vi "example_02_xy_graph_scrollbar.vi"() -> ()   [LabVIEW 2015, in "lv-graph.lvlib"]
doc: "This example will generate a fixed number of points, and then allow navigation of the data using the hofizontal and vertical scrollbar. You can configure the data rate (how often data is generated) and the refresh rate (how often the graphs update). This is a working example of how to separate data generation from display."
uses:
  advanced/build_graph-single_axis.vi
  advanced/build_graph-vertical.vi
  lv-graph.lvlib
panel:
  in  "vertical_scrollbar":i32(c297)
  out "vertical_graph":T1(graph)
  in  "refresh":bool
  in  "Flipped?":bool
  in  "# of Points to Generate":i32=5000
  in  "Realtime?":bool
  out "all_points_generated":bool
  in  "horizontal_scrollbar":i32(c297)
  in  "data_rate_ms":u32=10
  in  "refresh_rate_ms":i32=250
  in  "stop":bool
  out "horizontal_graph":T2(graph)
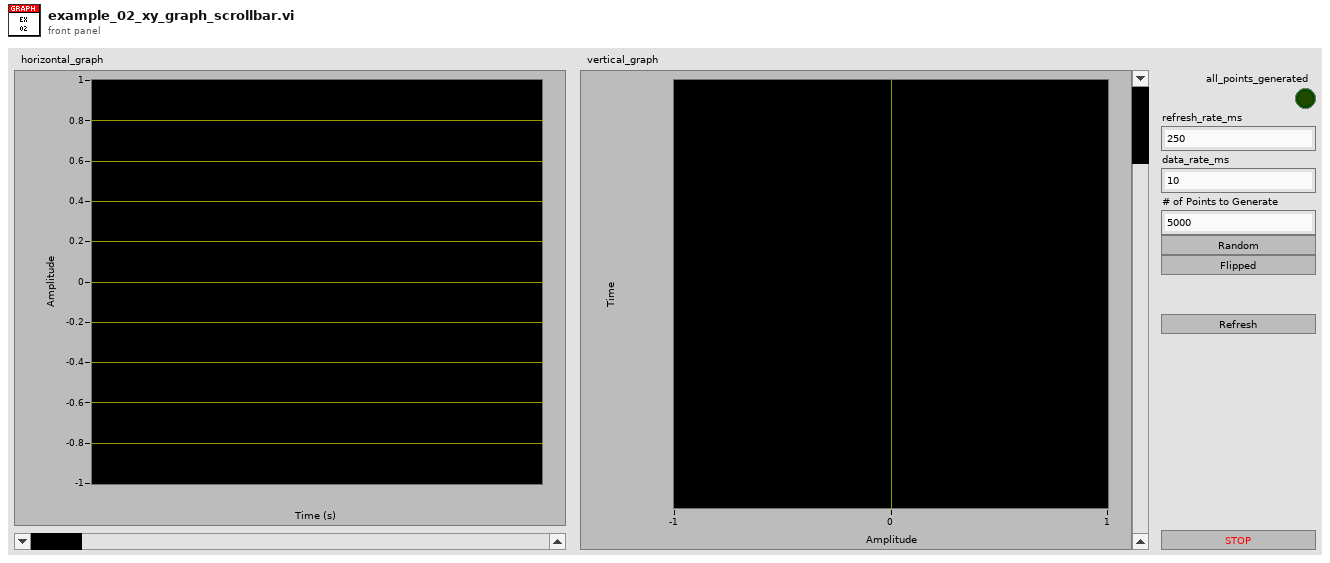
[diagram p1: front panel]
types:
  T1 = cluster{cluster{"Timestamp":dbl, "Timestamp":dbl}[]}[]
  T2 = cluster{"Time [] out":dbl[], "Data[][] out":dbl[]}[]
  T3 = cluster{"index":i32, "x_axis":dbl[], "y_axis":dbl[][]}
  T4 = cluster{"x_scale_maximum":dbl, "x_scale_minimum":dbl, "y_scale_maximum":dbl, "y_scale_minimum":dbl}
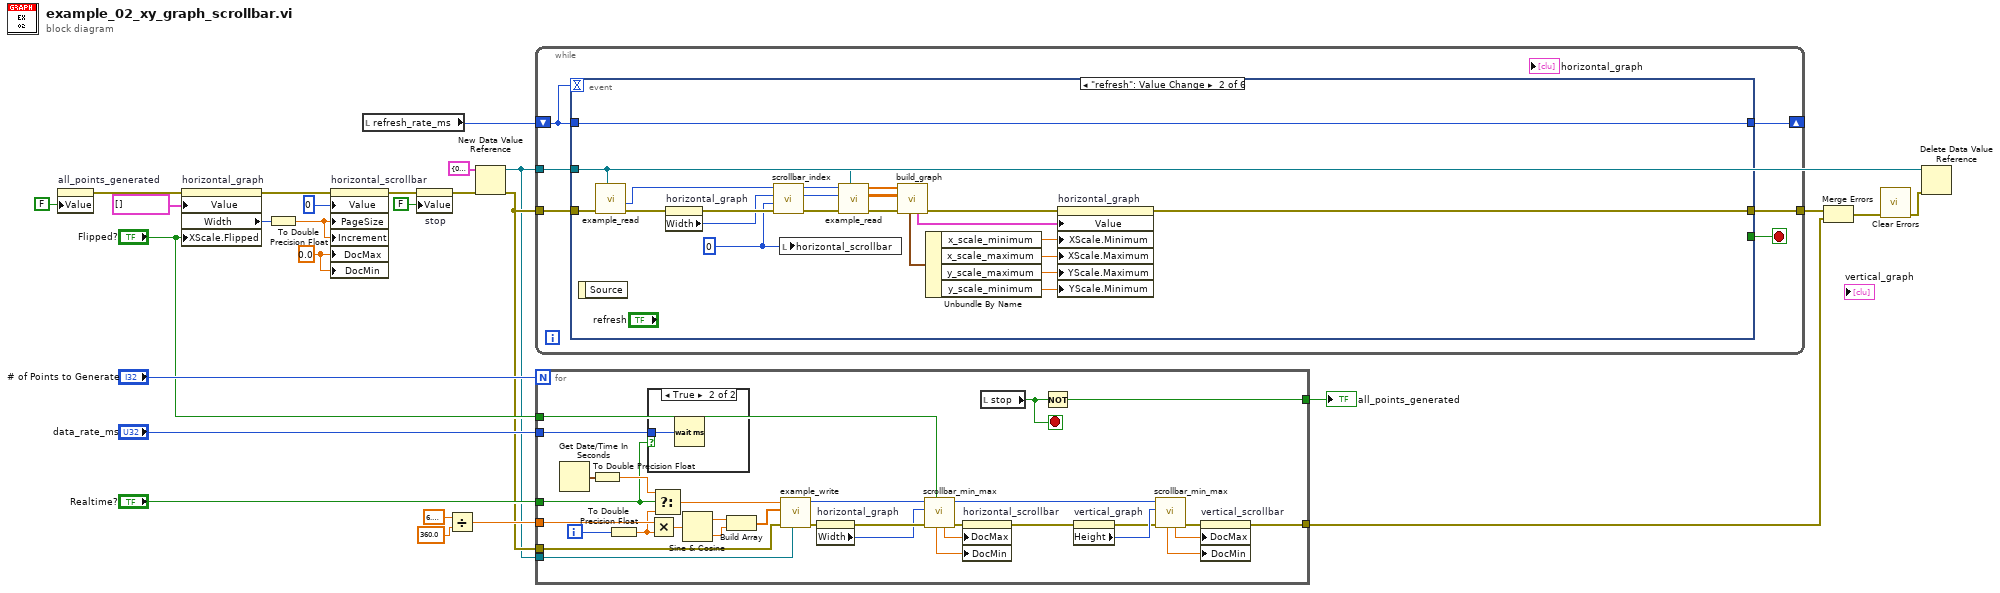
[diagram p0: block diagram]
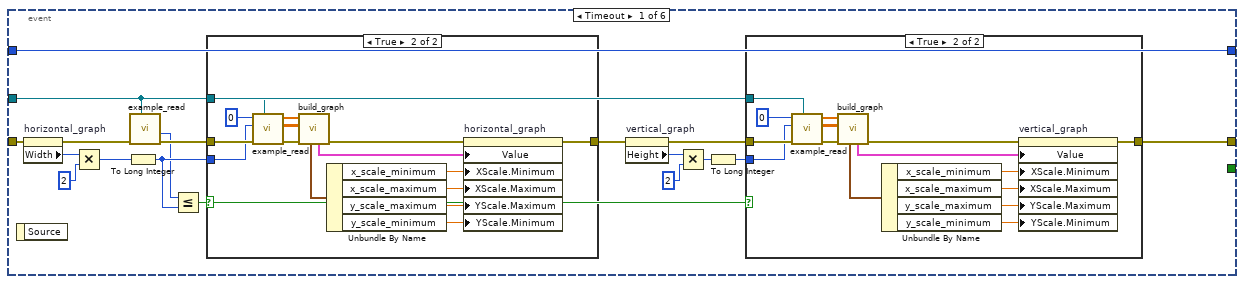
[diagram p2: hidden frame]
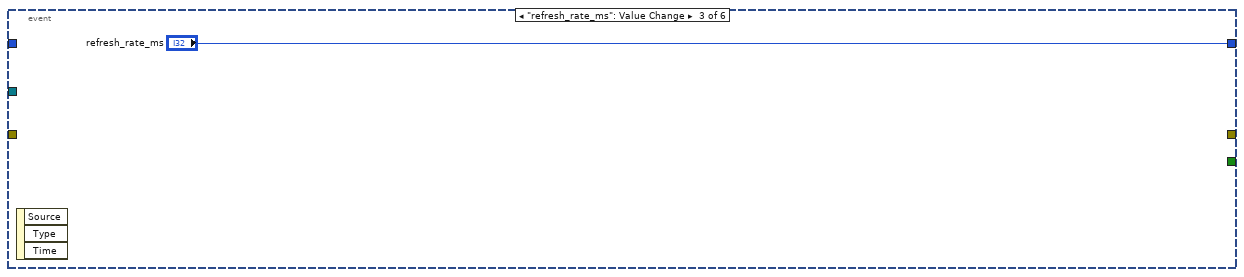
[diagram p5: hidden frame]
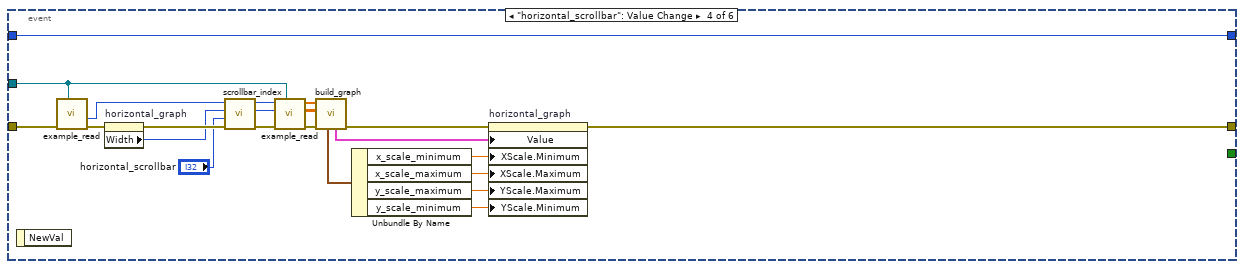
[diagram p6: hidden frame]
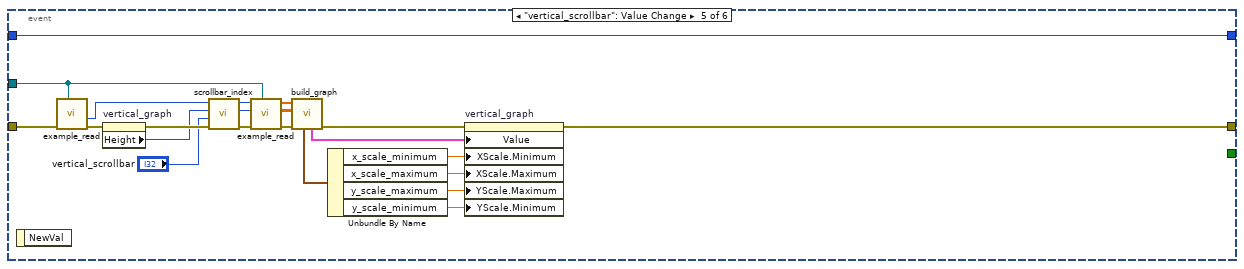
[diagram p7: hidden frame]
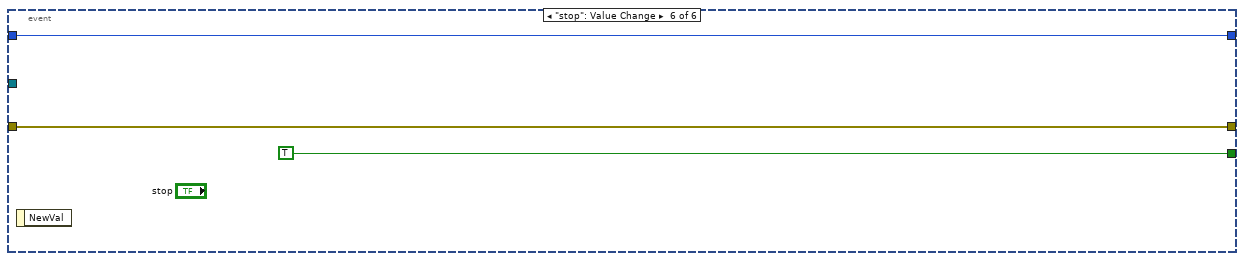
[diagram p8: hidden frame]
diagram:
  w18 = 0.0 ("Doc Max")
  n1 = property on="all_points_generated" class="Bool (strict)"("Value"=FALSE ("All Points Generated?")) -> (error out=w8:errorcluster)  [unwired: 2 in, 1 out]
  n2 = property on="horizontal_graph" class="XYGraph (strict)"(error in=w8, "Value"=T2 [] ("Graph"), "XScale.Flipped"="Flipped?") -> (error out=w19:errorcluster, "Width"=w17:u32)  [unwired: 1 in, 1 out]
  n3 = To Double Precision Float(number=w17) -> (double precision float=w6:dbl)
  n4 = property on="horizontal_scrollbar" class="Scroll (strict)"(error in=w19, "Value"=0 ("Scrollbar"), "PageSize"=w6, "Increment"=w6, "DocMax"=w18, "DocMin"=w18) -> (error out=w20:errorcluster)  [unwired: 1 in, 1 out]
  n5 = local read "refresh_rate_ms"() -> (w4:i32)
  n6 = property on="stop" class="Bool (strict)"(error in=w20, "Value"=FALSE ("Stop")) -> (error out=w26:errorcluster)  [unwired: 1 in, 1 out]
  n7 = Divide(x=6.283185307179586, y=360.0) -> (x/y=w12:dbl)
  n8 = New Data Value Reference(data value=T3 {"index"=0, "x_axis"=[], "y_axis"=[]} ("cluster"), error in=w26) -> (data value reference=w1:refnum<data-value>, error out=w3:errorcluster)
  n9 = while {
    tunnel: w3 -> [w33]
    tunnel: [w31] -> w25
    tunnel: w1 -> [w30]
    shift-right: [w28] -> _
    shift-left: w4 -> [w29]
    stop <- w32 stop-if-true
    n10 = event shown="[1] \"refresh\": Value Change" {
      selector: _ -> [_ _ _ _ _ _]
      dyn-events: _ -> [_ _ _ _ _ _]
      timeout: w29 -> [_ _ _ _ _ _]
      tunnel: w33 -> [w49 w101 _ w124 w146 w152]
      tunnel: [_ _ _ _ _ TRUE] -> w32
      tunnel: [w38 w105 _ w123 w145 w152] -> w31
      tunnel: w30 -> [w37 w94 _ w117 w140 _]
      tunnel: w29 -> [w44 w95 _ w119 w141 w151]
      tunnel: [w44 w95 "refresh_rate_ms" w119 w141 w151] -> w28
      event Timeout {
        n11 = event-data() -> ()  [unwired: 1 in, 1 out]
        n12 = property on="horizontal_graph" class="XYGraph (strict)"(error in=w49) -> (error out=w47:errorcluster, "Width"=w50:u32)  [unwired: 1 in, 1 out]
        n13 = Multiply(x=w50, y=u32 2 ("x")) -> (x*y=w48:u32)
        n14 = To Long Integer(number=w48) -> (32bit integer=w45:i32)
        n15 = call "example_read.vi"("dvr"=w37, "error in (no error)"=w47) -> ("error out"=w46:errorcluster, "index"=w35:i32)  [unwired: 6 in, 2 out]
        n16 = Less Or Equal?(x=w35, y=w45) -> (x <= y?=w34:bool)
        n17 = case shown="True" w34 {
          tunnel: w46 -> [w68 w78]
          tunnel: [w68 w75] -> w39
          tunnel: w45 -> [_ w73]
          tunnel: w37 -> [_ w76]
          frame False {
          }
          frame True {
            n18 = call "example_read.vi"("dvr"=w76, "error in (no error)"=w78, "length"=w73, "index in"=0 ("Index in")) -> ("error out"=w77:errorcluster, "y_axis"=w71:dbl[][], "x_axis"=w72:dbl[])  [unwired: 4 in, 1 out]
            n19 = call-poly "build_graph.vi"("error in (no error)"=w77, "y_axis"=w71, "x_axis"=w72) -> ("error out"=w83:errorcluster, "graph_data"=w69:cluster{dbl[], dbl[]}[], "scale_ranges"=w70:T4)  [unwired: 6 in]
            n20 = Unbundle By Name(w70) -> ("x_scale_minimum"=w81:dbl, "x_scale_maximum"=w82:dbl, "y_scale_maximum"=w80:dbl, "y_scale_minimum"=w79:dbl)
            n21 = property on="horizontal_graph" class="XYGraph (strict)"(error in=w83, "Value"=w69, "XScale.Minimum"=w81, "XScale.Maximum"=w82, "YScale.Maximum"=w80, "YScale.Minimum"=w79) -> (error out=w75:errorcluster)  [unwired: 1 in, 1 out]
          }
        }
        n22 = property on="vertical_graph" class="XYGraph (strict)"(error in=w39) -> (error out=w36:errorcluster, "Height"=w41:u32)  [unwired: 1 in, 1 out]
        n23 = Multiply(x=w41, y=u32 2 ("x")) -> (x*y=w42:u32)
        n24 = To Long Integer(number=w42) -> (32bit integer=w43:i32)
        n25 = case shown="True" w34 {
          tunnel: w36 -> [w52 w66]
          tunnel: [w52 w63] -> w38
          tunnel: w43 -> [_ w61]
          tunnel: w37 -> [_ w60]
          frame False {
          }
          frame True {
            n26 = call "example_read.vi"("dvr"=w60, "error in (no error)"=w66, "length"=w61, "index in"=0 ("Index in")) -> ("error out"=w65:errorcluster, "y_axis"=w64:dbl[][], "x_axis"=w59:dbl[])  [unwired: 4 in, 1 out]
            n27 = call-poly "build_graph.vi"("error in (no error)"=w65, "y_axis"=w64, "x_axis"=w59) -> ("error out"=w67:errorcluster, "graph_data"=w57:T1, "scale_ranges"=w58:T4)  [unwired: 6 in]
            n28 = Unbundle By Name(w58) -> ("x_scale_minimum"=w56:dbl, "x_scale_maximum"=w55:dbl, "y_scale_maximum"=w54:dbl, "y_scale_minimum"=w53:dbl)
            n29 = property on="vertical_graph" class="XYGraph (strict)"(error in=w67, "Value"=w57, "XScale.Minimum"=w56, "XScale.Maximum"=w55, "YScale.Maximum"=w54, "YScale.Minimum"=w53) -> (error out=w63:errorcluster)  [unwired: 1 in, 1 out]
          }
        }
      }
      event "refresh": Value Change {
        w100 = 0 ("Seek")
        n30 = event-data() -> ()  [unwired: 1 in, 1 out]
        n31 = call "example_read.vi"("dvr"=w94, "error in (no error)"=w101) -> ("error out"=w102:errorcluster, "index"=w88:i32)  [unwired: 6 in, 2 out]
        n32 = property on="horizontal_graph" class="XYGraph (strict)"(error in=w102) -> (error out=w104:errorcluster, "Width"=w103:u32)  [unwired: 1 in, 1 out]
        n33 = call "scrollbar_index.vi"("error in (no error)"=w104, "seek"=w100, "width_height"=w103, "data_available"=w88) -> ("error out"=w96:errorcluster, "length"=w89:i32, "index"=w90:i32)  [unwired: 5 in]
        n34 = local write "horizontal_scrollbar"(w100) -> ()
        n35 = call "example_read.vi"("dvr"=w94, "error in (no error)"=w96, "length"=w89, "index in"=w90) -> ("error out"=w97:errorcluster, "y_axis"=w98:dbl[][], "x_axis"=w91:dbl[])  [unwired: 4 in, 1 out]
        n36 = call-poly "build_graph.vi"("error in (no error)"=w97, "y_axis"=w98, "x_axis"=w91) -> ("error out"=w99:errorcluster, "graph_data"=w92:cluster{dbl[], dbl[]}[], "scale_ranges"=w93:T4)  [unwired: 6 in]
        n37 = Unbundle By Name(w93) -> ("x_scale_minimum"=w87:dbl, "x_scale_maximum"=w86:dbl, "y_scale_maximum"=w85:dbl, "y_scale_minimum"=w84:dbl)
        n38 = property on="horizontal_graph" class="XYGraph (strict)"(error in=w99, "Value"=w92, "XScale.Minimum"=w87, "XScale.Maximum"=w86, "YScale.Maximum"=w85, "YScale.Minimum"=w84) -> (error out=w105:errorcluster)  [unwired: 1 in, 1 out]
      }
      event "refresh_rate_ms": Value Change {
        n39 = event-data() -> ()  [unwired: 1 in, 3 out]
      }
      event "horizontal_scrollbar": Value Change {
        n40 = event-data() -> ()  [unwired: 1 in, 1 out]
        n41 = call "example_read.vi"("dvr"=w117, "error in (no error)"=w124) -> ("error out"=w125:errorcluster, "index"=w116:i32)  [unwired: 6 in, 2 out]
        n42 = property on="horizontal_graph" class="XYGraph (strict)"(error in=w125) -> (error out=w128:errorcluster, "Width"=w126:u32)  [unwired: 1 in, 1 out]
        n43 = call "scrollbar_index.vi"("error in (no error)"=w128, "seek"="horizontal_scrollbar", "width_height"=w126, "data_available"=w116) -> ("error out"=w120:errorcluster, "length"=w114:i32, "index"=w115:i32)  [unwired: 5 in]
        n44 = call "example_read.vi"("dvr"=w117, "error in (no error)"=w120, "length"=w114, "index in"=w115) -> ("error out"=w121:errorcluster, "y_axis"=w122:dbl[][], "x_axis"=w113:dbl[])  [unwired: 4 in, 1 out]
        n45 = call-poly "build_graph.vi"("error in (no error)"=w121, "y_axis"=w122, "x_axis"=w113) -> ("error out"=w127:errorcluster, "graph_data"=w111:cluster{dbl[], dbl[]}[], "scale_ranges"=w112:T4)  [unwired: 6 in]
        n46 = Unbundle By Name(w112) -> ("x_scale_minimum"=w110:dbl, "x_scale_maximum"=w109:dbl, "y_scale_maximum"=w108:dbl, "y_scale_minimum"=w107:dbl)
        n47 = property on="horizontal_graph" class="XYGraph (strict)"(error in=w127, "Value"=w111, "XScale.Minimum"=w110, "XScale.Maximum"=w109, "YScale.Maximum"=w108, "YScale.Minimum"=w107) -> (error out=w123:errorcluster)  [unwired: 1 in, 1 out]
      }
      event "vertical_scrollbar": Value Change {
        n48 = event-data() -> ()  [unwired: 1 in, 1 out]
        n49 = call "example_read.vi"("dvr"=w140, "error in (no error)"=w146) -> ("error out"=w147:errorcluster, "index"=w129:i32)  [unwired: 6 in, 2 out]
        n50 = property on="vertical_graph" class="XYGraph (strict)"(error in=w147) -> (error out=w150:errorcluster, "Height"=w148:u32)  [unwired: 1 in, 1 out]
        n51 = call "scrollbar_index.vi"("error in (no error)"=w150, "seek"="vertical_scrollbar", "width_height"=w148, "data_available"=w129) -> ("error out"=w142:errorcluster, "length"=w130:i32, "index"=w131:i32)  [unwired: 5 in]
        n52 = call "example_read.vi"("dvr"=w140, "error in (no error)"=w142, "length"=w130, "index in"=w131) -> ("error out"=w143:errorcluster, "y_axis"=w144:dbl[][], "x_axis"=w132:dbl[])  [unwired: 4 in, 1 out]
        n53 = call-poly "build_graph.vi"("error in (no error)"=w143, "y_axis"=w144, "x_axis"=w132) -> ("error out"=w149:errorcluster, "graph_data"=w137:T1, "scale_ranges"=w138:T4)  [unwired: 6 in]
        n54 = Unbundle By Name(w138) -> ("x_scale_minimum"=w136:dbl, "x_scale_maximum"=w135:dbl, "y_scale_maximum"=w134:dbl, "y_scale_minimum"=w133:dbl)
        n55 = property on="vertical_graph" class="XYGraph (strict)"(error in=w149, "Value"=w137, "XScale.Minimum"=w136, "XScale.Maximum"=w135, "YScale.Maximum"=w134, "YScale.Minimum"=w133) -> (error out=w145:errorcluster)  [unwired: 1 in, 1 out]
      }
      event "stop": Value Change {
        n56 = event-data() -> ()  [unwired: 1 in, 1 out]
      }
    }
  }
  n57 = for {
    N: "# of Points to Generate" -> [_]
    tunnel: w12 -> [w182]
    tunnel: "Realtime?" -> [w169]
    tunnel: "data_rate_ms" -> [w170]
    tunnel: [w175] -> w15
    tunnel: "Flipped?" -> [w171]
    tunnel: w3 -> [w168]
    tunnel: [w159] -> w9
    tunnel: w1 -> [w164]
    i -> [w183]
    stop <- w176 stop-if-true
    n58 = Get Date/Time In Seconds() -> (seconds since 1Jan1904=w184:timestamp)
    n59 = To Double Precision Float(number=w184) -> (double precision float=w181:dbl)
    n60 = To Double Precision Float(number=w183) -> (double precision float=w180:dbl)
    n61 = case shown="True" w169 {
      tunnel: w170 -> [_ w185]
      frame False {
      }
      frame True {
        n62 = Wait (ms)(milliseconds to wait=w185) -> ()  [unwired: 1 out]
      }
    }
    n63 = Multiply(x=w182, y=w180) -> (x*y=w179:dbl)
    n64 = Select(t=w181, s=w169, f=w180) -> (s? t:f=w166:dbl)
    n65 = Sine & Cosine(0:w179) -> (1:w178:dbl, 2:w177:dbl)
    n66 = Build Array(w178, w177) -> (w165:dbl[])
    n67 = call "example_write.vi"("dvr"=w164, "error in (no error)"=w168, "y_axis"=w165, "x_axis"=w166) -> ("error out"=w167:errorcluster, "index"=w158:i32)  [unwired: 6 in]
    n68 = property on="horizontal_graph" class="XYGraph (strict)"(error in=w167) -> (error out=w173:errorcluster, "Width"=w172:u32)  [unwired: 1 in, 1 out]
    n69 = call "scrollbar_min_max.vi"("flipped"=w171, "error in (no error)"=w173, "width_height"=w172, "data_index in"=w158) -> ("error out"=w174:errorcluster, "scrollbar_doc_max"=w157:dbl, "scrollbar_doc_min"=w156:dbl)  [unwired: 5 in]
    n70 = property on="horizontal_scrollbar" class="Scroll (strict)"(error in=w174, "DocMax"=w157, "DocMin"=w156) -> (error out=w160:errorcluster)  [unwired: 1 in, 1 out]
    n71 = local read "stop"() -> (w176:bool)
    n72 = Not(x=w176) -> (.not. x?=w175:bool)
    n73 = property on="vertical_graph" class="XYGraph (strict)"(error in=w160) -> (error out=w162:errorcluster, "Height"=w163:u32)  [unwired: 1 in, 1 out]
    n74 = call "scrollbar_min_max.vi"("error in (no error)"=w162, "width_height"=w163, "data_index in"=w158) -> ("error out"=w161:errorcluster, "scrollbar_doc_max"=w155:dbl, "scrollbar_doc_min"=w154:dbl)  [unwired: 6 in]
    n75 = property on="vertical_scrollbar" class="Scroll (strict)"(error in=w161, "DocMax"=w155, "DocMin"=w154) -> (error out=w159:errorcluster)  [unwired: 1 in, 1 out]
  }
  "all_points_generated" <- w15
  n76 = Merge Errors(w25, w9) -> (w5:errorcluster)
  n77 = call <vilib>:"Clear Errors.vi"("error in (no error)"=w5) -> ("error out"=w27:errorcluster)  [unwired: 5 in, 1 out]
  n78 = Delete Data Value Reference(data value reference=w1, error in=w27) -> ()  [unwired: 2 out]
